vi "Configure Temperature.vi"(8 "error in (no error)":errorcluster, 10 "Temp Scale":u16(ring)=1 items=["C", "F"], 11 "VISA resource name":refnum<visa-resource-name>) -> (0 "error out":errorcluster, 1 "concatenated string":string, 3 "VISA resource name out":refnum<visa-resource-name>)   [LabVIEW 2013, in "Fluke 2625A.lvlib"]
uses:
  <instrlib>/Fluke 2625A/Fluke 2625A.lvlib
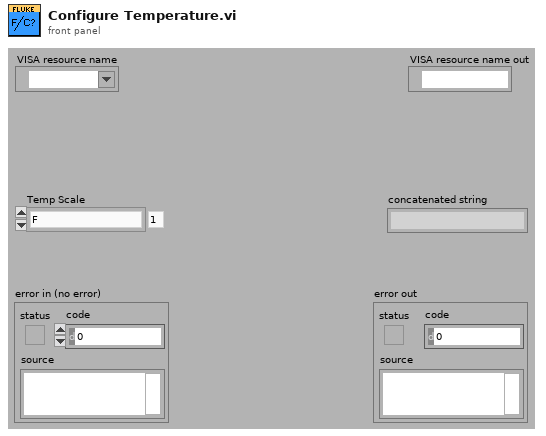
[diagram p1: front panel]
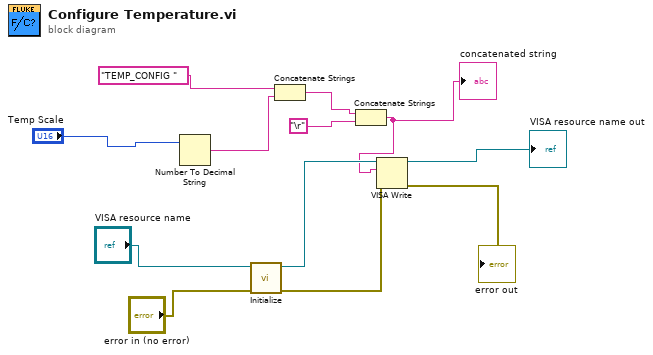
[diagram p0: block diagram]
diagram:
  n1 = Number To Decimal String(number="Temp Scale") -> (decimal integer string=w11:string)  [unwired: 1 in]
  n2 = call <instrlib>:"Initialize.vi"("error In"="error in (no error)", "VISA resource name"="VISA resource name") -> ("error out"=w5:errorcluster, "VISA resource name out"=w7:refnum<visa-resource-name>)  [unwired: 7 in, 1 out]
  n3 = Concatenate Strings("TEMP_CONFIG ", w11) -> (w2:string)
  n4 = Concatenate Strings(w2, "\r") -> (w1:string)
  "concatenated string" <- w1
  n5 = VISA Write(VISA resource name=w7, write buffer=w1, error in (no error)=w5) -> (VISA resource name out=→"VISA resource name out":refnum<visa-resource-name>, error out=→"error out":errorcluster)  [unwired: 1 out]
